vi "Read Mfg Serial Number.vi"(8 "error in":errorcluster) -> (0 "error out":errorcluster, 3 "Serial Number":string)   [LabVIEW 2015]
uses:
  CAN Communication/PAS/PAS.lvclass
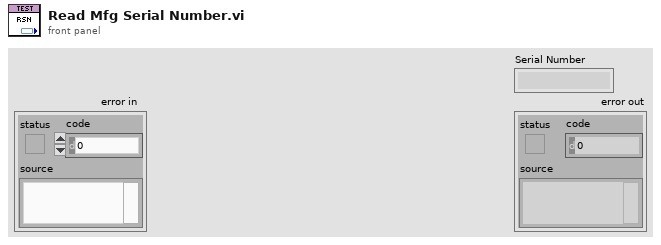
[diagram p1: front panel]
types:
  T1 = typedef "PAS.lvclass/Session Handle.ctl" = refnum<data-value>
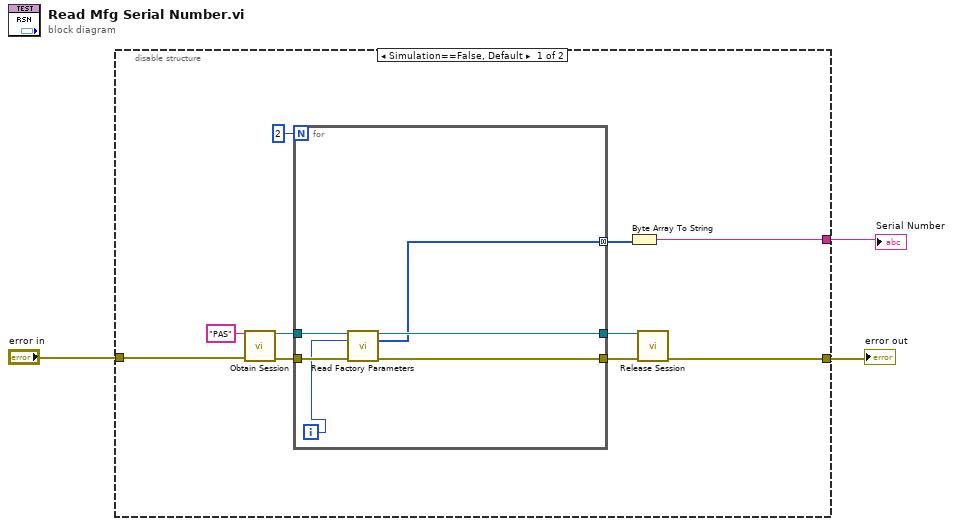
[diagram p0: block diagram]
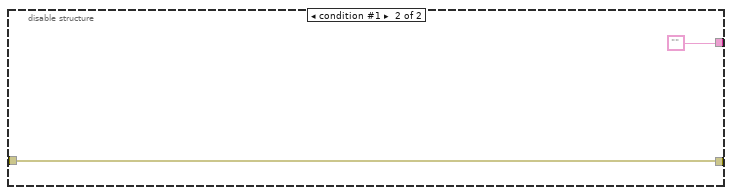
[diagram p2: hidden frame]
diagram:
  n1 = disable-structure shown="Simulation==False, Default" {
    disable-tunnel: [w7 w21] -> w3
    disable-tunnel: "error in" -> [w6 w21]
    disable-tunnel: [w5 ""] -> w1
    frame condition #0 (active) {
      n2 = call "Obtain Session.vi"("Session  Name ()"="PAS", "error in (no error)"=w6) -> ("Session Handle"=w13:T1, "error out"=w12:errorcluster)  [unwired: 12 in]
      n3 = for {
        N: 2 -> [_]
        tunnel: w13 -> [w19]
        tunnel: w12 -> [w18]
        tunnel: [w16] -> w10
        tunnel: [w15] -> w9
        tunnel: [w14] -> w8 mode=concatenating
        i -> [w17]
        n4 = call "Read Factory Parameters.vi"("Session Handle in"=w19, "Address"=w17, "error in (no error)"=w18) -> ("Session Handle out"=w16:T1, "Read Bytes"=w14:u8[], "error out"=w15:errorcluster)  [unwired: 10 in]
      }
      n5 = Byte Array To String(unsigned byte array=w8) -> (string=w5:string)
      n6 = call "Release Session.vi"("Session Handle"=w10, "error in (no error)"=w9) -> ("error out"=w7:errorcluster)  [unwired: 13 in]
    }
    frame condition #1 {
    }
  }
  "error out" <- w3
  "Serial Number" <- w1
